vi "XLP80_EA_WriteOutputs_Batterie.vi"(8 "err in":errorcluster, 11 "Device information":string[](array[string])=["ASRL1::INSTR", "EL 3160-60 A", "000", "///", "1", "160", "60", "400", "10", "400"]) -> (0 "err out":errorcluster, 3 "Device information IN":string[](array[string])=["ASRL1::INSTR", "EL 3160-60 A", "000", "///", "1", "160", "60", "400", "10", "400"])   [LabVIEW 2021]
uses:
  XLP80_EA_Globals.vi
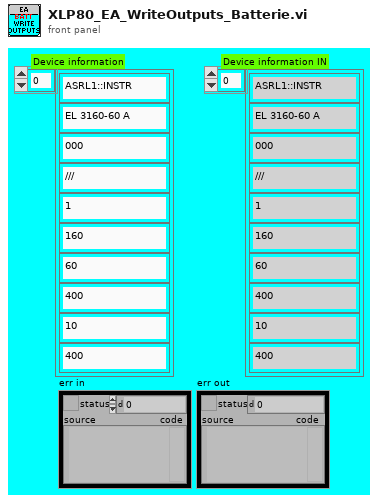
[diagram p1: front panel]
types:
  T1 = typedef "XLP80_EA_TDefsCluster_EA Setpoint.ctl" = cluster{"Load":bool, "Set Current":sgl, "Set Voltage":sgl}
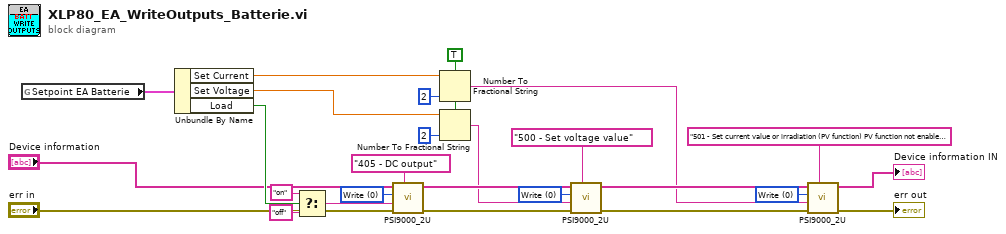
[diagram p0: block diagram]
diagram:
  w4 = u8 0 items=["Write", "Read"] ("Access")
  w5 = u8 0 items=["Write", "Read"] ("Access")
  w2 = TRUE ("use system decimal point (T)")
  w20 = u8 0 items=["Write", "Read"] ("Access")
  n1 = global read "XLP80_EA_Globals.vi" "Setpoint EA Batterie"() -> (w26:T1)
  n2 = Unbundle By Name(w26) -> ("Set Current"=w1:sgl, "Set Voltage"=w21:sgl, "Load"=w25:bool)
  n3 = Select(t="on" ("Value"), s=w25, f="off") -> (s? t:f=w18:string)
  n4 = call <instrlib>:"PSI9000_2U.vi"("Command list"="405 - DC output", "Error in"="err in", "Value"=w18, "Access"=w20, "Device information in"="Device information") -> ("Error out"=w12:errorcluster, "Device information out"=w13:string[])  [unwired: 1 in, 2 out]
  n5 = Number To Fractional String(use system decimal point (T)=w2, number=w1, precision (6)=i16 2) -> (F-format string=w7:string)  [unwired: 1 in]
  n6 = Number To Fractional String(use system decimal point (T)=w2, number=w21, precision (6)=i16 2) -> (F-format string=w9:string)  [unwired: 1 in]
  n7 = call <instrlib>:"PSI9000_2U.vi"("Command list"="500 - Set voltage value", "Error in"=w12, "Value"=w9, "Access"=w5, "Device information in"=w13) -> ("Error out"=w11:errorcluster, "Device information out"=w10:string[])  [unwired: 1 in, 2 out]
  n8 = call <instrlib>:"PSI9000_2U.vi"("Command list"="501 - Set current value or irradiation (PV function) PV function not enabled for PSB/PSBEE PSB/PSBE 9000: source mode", "Error in"=w11, "Value"=w7, "Access"=w4, "Device information in"=w10) -> ("Error out"=→"err out":errorcluster, "Device information out"=→"Device information IN":string[])  [unwired: 1 in, 2 out]
